vi "Autofocus-Broken.vi"(0 "controller in":refnum<k24>, 1 "AbortAutoFocus":bool, 5 "SafeMaxZ":dbl=86.0 format="%#_13g", 7 "InitialStepSize":dbl=0.1, 9 "Tolerance":dbl=0.005 format="%#_13g", 11 "error in (no error)":errorcluster) -> (4 "controller out":refnum<k24>, 6 "Image":T2(plugin-control), 8 "N_iterations":dbl, 10 "BestZvalue":dbl, 15 "error out":errorcluster)   [LabVIEW 2019]
uses:
  <vilib>/vision/NI_Vision_Development_Module.lvlib
  <vilib>/vision/driver/NI_Vision_Acquisition_Software.lvlib
  <vilib>/vision/driver/IMAQdx.llb/IMAQdx Buffer Number Mode.ctl
  <vilib>/Utility/error.llb/DialogType.ctl
  C:/Users/TTUHEP/Documents/LabVIEW/Other Models/2010/Bin/Aerotech.A3200.dll
  Other Models/2010/Bin/Aerotech.A3200.dll
  <vilib>/userDefined/High Color/IMAQdx.ctl
panel:
  out "ZvsSD":string
  in  "Camera":T1="cam1"
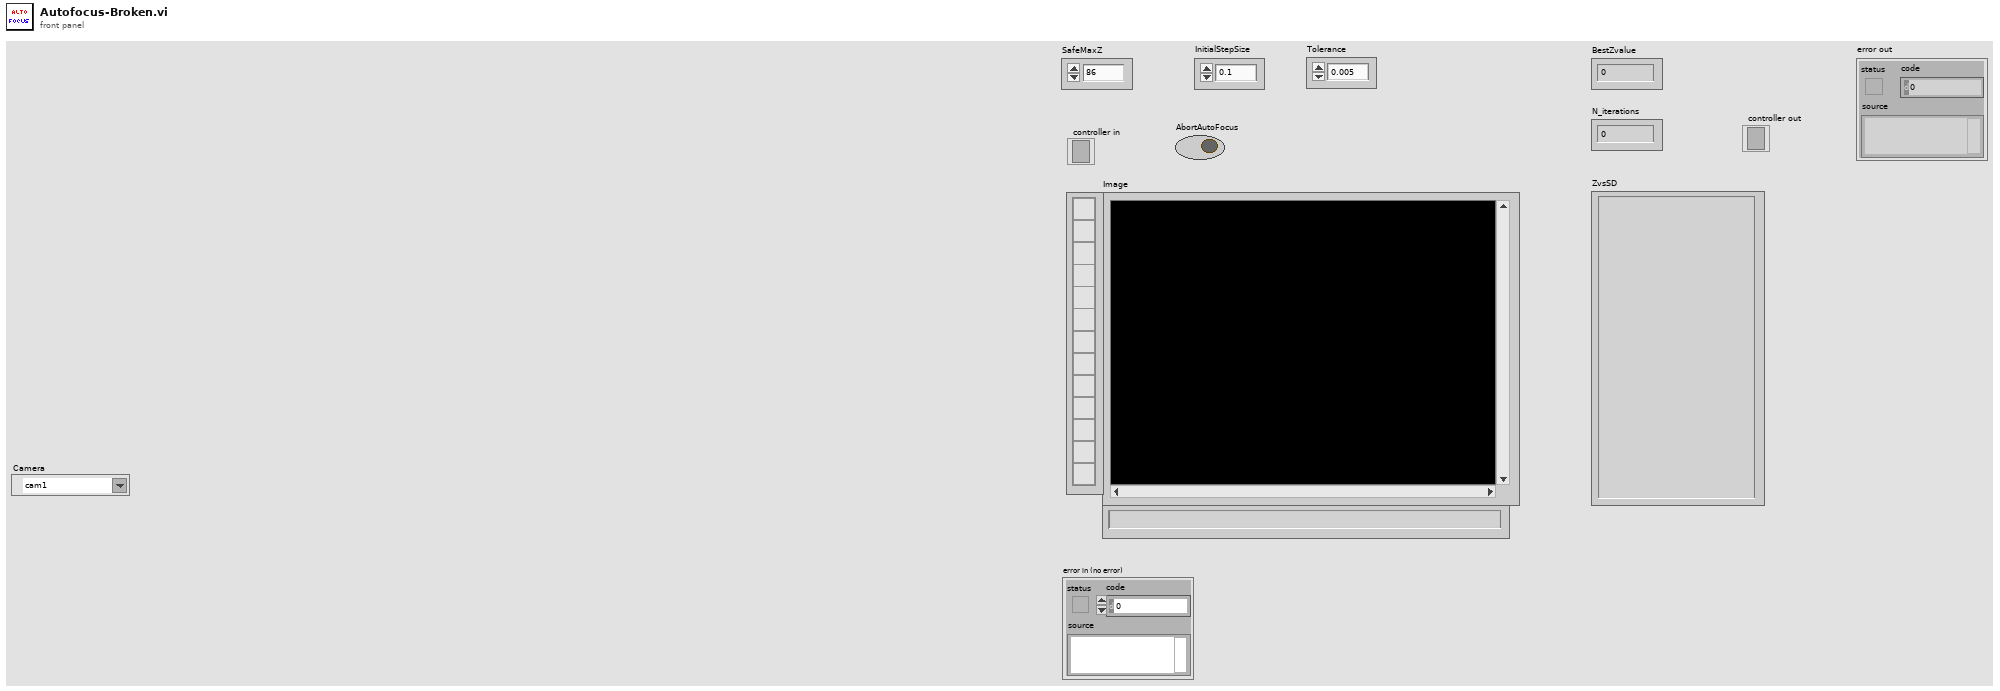
[diagram p1: front panel]
types:
  T1 = typedef "IMAQdx.ctl" = refnum<k21>
  T2 = typedef "IMAQ Image.ctl" = refnum<image>
  T3 = typedef "Image Type" = u32
  T4 = enum32{"Differentiation", "Gradient", "Prewitt", "Roberts", "Sigma", "Sobel"}
  T5 = typedef "NI_Vision_Acquisition_Software.lvlib/IMAQdx Buffer Number Mode.ctl" = enum32{"Next", "Last", "Buffer Number", "Every", "Last New"}
  T6 = typedef "DialogType.ctl" = u16
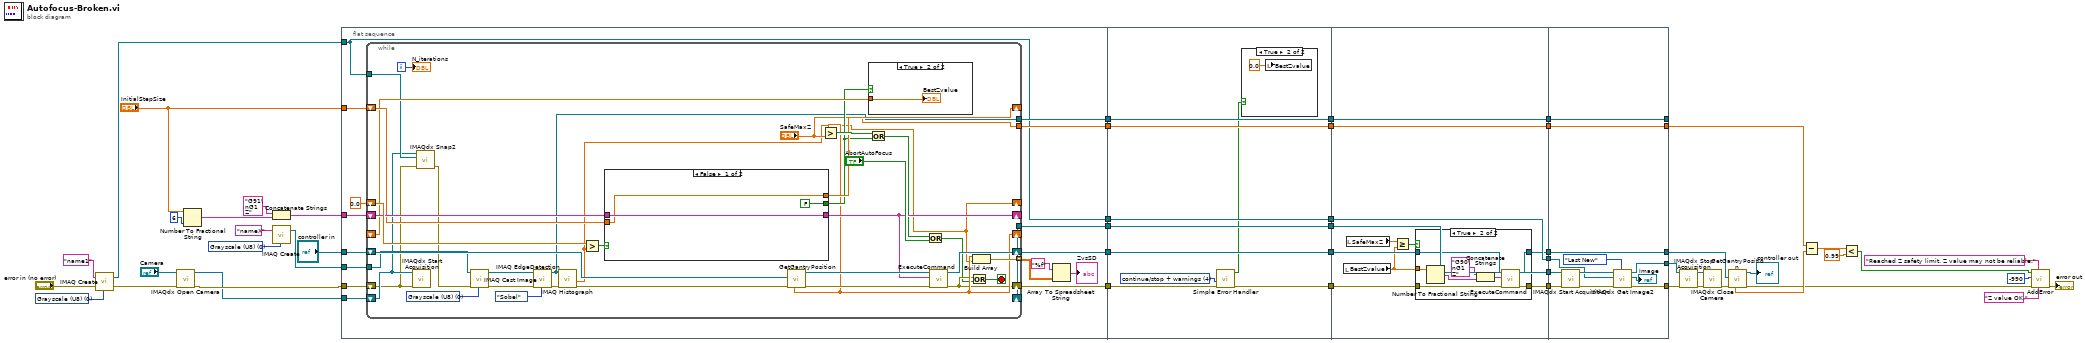
[diagram p0: block diagram]
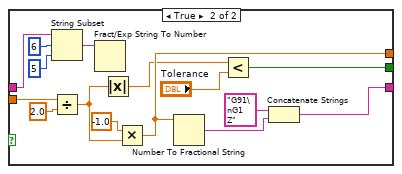
[diagram p3: hidden frame]
diagram:
  w26 = T3 0 items=["Grayscale (U8)", "Grayscale (I16)", "Grayscale (SGL)", "Complex (CSG)", "RGB (U32)", "HSL (U32)", "RGB (U64)", "Grayscale (U16)"] ("Image Type")
  w29 = T3 0 items=["Grayscale (U8)", "Grayscale (I16)", "Grayscale (SGL)", "Complex (CSG)", "RGB (U32)", "HSL (U32)", "RGB (U64)", "Grayscale (U16)"] ("Image Type")
  n1 = call "IMAQ Create"("Image Name"="name1" ("ImageName"), "Image Type"=w29, "error in (no error)"="error in (no error)") -> ("New Image"=w28:T2, "error out"=w31:errorcluster)  [unwired: 2 in]
  n2 = call <vilib>:"IMAQdx Open Camera.vi"("error in"=w31, "Session In"="Camera") -> ("error out"=w18:errorcluster, "Session Out"=w17:T1)  [unwired: 8 in]
  n3 = Number To Fractional String(number="InitialStepSize", precision (6)=i16 6) -> (F-format string=w47:string)  [unwired: 2 in]
  n4 = Concatenate Strings("G91\nG1 Z", w47) -> (w49:string)
  n5 = call "IMAQ Create"("Image Name"="nameX", "Image Type"=w26) -> ("New Image"=w13:T2)  [unwired: 3 in, 1 out]
  n6 = flat-sequence {
    tunnel: "controller in" -> [w68]
    tunnel: "InitialStepSize" -> [w66]
    tunnel: w49 -> [w65]
    tunnel: w18 -> [w64]
    tunnel: [w63] -> w12
    tunnel: [w62] -> w10
    tunnel: [w61] -> w8
    tunnel: [w60] -> w6
    tunnel: [w58] -> w4
    tunnel: w17 -> [w59]
    tunnel: w28 -> [w53]
    tunnel: [w53] -> w2
    tunnel: w13 -> [w54]
    tunnel: w12 -> [w132]
    tunnel: [w132] -> w11
    tunnel: w10 -> [w131]
    tunnel: [w131] -> w9
    tunnel: w8 -> [w127]
    tunnel: [w126] -> w7
    tunnel: w6 -> [w130]
    tunnel: [w130] -> w5
    tunnel: w4 -> [w129]
    tunnel: [w129] -> w3
    tunnel: w2 -> [w128]
    tunnel: [w128] -> w1
    tunnel: w11 -> [w140]
    tunnel: [w137] -> w24
    tunnel: w9 -> [w144]
    tunnel: [w144] -> w23
    tunnel: w7 -> [w139]
    tunnel: [w138] -> w22
    tunnel: w5 -> [w143]
    tunnel: [w143] -> w21
    tunnel: w3 -> [w142]
    tunnel: [w142] -> w20
    tunnel: w1 -> [w141]
    tunnel: [w141] -> w19
    tunnel: [w164] -> _
    tunnel: [w165] -> w35
    tunnel: [w166] -> w46
    tunnel: w24 -> [w166]
    tunnel: w23 -> [w165]
    tunnel: w22 -> [w156]
    tunnel: w21 -> [w164]
    tunnel: [w155] -> w34
    tunnel: [w158] -> w33
    tunnel: w20 -> [w160]
    tunnel: w19 -> [w159]
    frame #0 {
      n7 = while {
        shift-right: [w98] -> w63
        shift-left: w68 -> [w101]
        shift-right: [w75] -> w61
        shift-left: w64 -> [w70]
        shift-right: [w95] -> _
        shift-left: w65 -> [w94]
        shift-right: [w78] -> _
        shift-left: 0.0 -> [w97]
        shift-right: [w91] -> _
        shift-left: w66 -> [w90]
        shift-right: [w79] -> _
        shift-left: _ -> [w89]
        tunnel: ["SafeMaxZ"] -> w62
        tunnel: [w83] -> w60
        tunnel: w54 -> [w77]
        tunnel: [w76] -> w58
        tunnel: [w80] -> w55 mode=indexing
        shift-right: [w76] -> _
        shift-left: w59 -> [w71]
        tunnel: w53 -> [w72]
        i -> [w86]
        stop <- w73 stop-if-true
        w87 = T3 0 items=["Grayscale (U8)", "Grayscale (I16)", "Grayscale (SGL)", "Complex (CSG)", "RGB (U32)", "HSL (U32)", "RGB (U64)", "Grayscale (U16)"] ("Image Type")
        n8 = call <vilib>:"IMAQdx Start Acquisition.vi"("error in"=w70, "Session In"=w71) -> ()  [unwired: 8 in, 2 out]
        n9 = call <vilib>:"IMAQdx Snap2.vi"("error in"=w70, "Image In"=w72, "Session In"=w71) -> ("error out"=w69:errorcluster)  [unwired: 6 in, 2 out]
        n10 = call "IMAQ Cast Image"("Image Type"=w87, "error in (no error)"=w69, "Image Src"=w77) -> ("error out"=w81:errorcluster, "Image Dst Out"=w102:T2)  [unwired: 7 in]
        n11 = call "IMAQ EdgeDetection"("Method"=T4."Sobel", "error in (no error)"=w81, "Image Src"=w102) -> ("error out"=w104:errorcluster, "Image Dst Out"=w83:T2)  [unwired: 7 in]
        n12 = call "IMAQ Histograph"("error in (no error)"=w104, "Image"=w83) -> ("error out"=w84:errorcluster, "Standard  Deviation"=w78:sgl)  [unwired: 6 in, 2 out]
        n13 = Greater?(x=w97, y=w78) -> (0:w96:bool)
        n14 = case shown="False" w96 {
          tunnel: [w108 w122] -> w95
          tunnel: w94 -> [w108 w116]
          tunnel: [FALSE w117] -> w88
          tunnel: [w106 w112] -> w91
          tunnel: w90 -> [w106 w111]
          frame False {
          }
          frame True {
            n15 = String Subset(string=w116, offset (0)=6, length (rest)=5) -> (substring=w113:string)
            n16 = Divide(x=w111, y=2.0) -> (x/y=w110:dbl)
            n17 = Fract/Exp String To Number(string=w113) -> ()  [unwired: 3 in, 2 out]
            n18 = Absolute Value(x=w110) -> (abs(x)=w109:dbl)
            n19 = Multiply(x=-1.0, y=w110) -> (x*y=w112:dbl)
            n20 = Number To Fractional String(number=w112) -> (F-format string=w121:string)  [unwired: 3 in]
            n21 = Less?(x=w109, y="Tolerance") -> (x < y?=w117:bool)
            n22 = Concatenate Strings("G91\nG1 Z", w121) -> (w122:string)
          }
        }
        n23 = call "GetGantryPosition.vi"("error in (no error)"=w84, "Controller In"=w101) -> ("error out"=w100:errorcluster, "controller out"=w99:refnum<k24>, "Position Z"=w79:dbl)  [unwired: 3 in, 4 out]
        n24 = Greater?(x=w79, y="SafeMaxZ") -> (0:w93:bool)
        n25 = case shown="True" w88 {
          tunnel: w89 -> [_ w105]
          frame False {
          }
          frame True {
            "BestZvalue" <- w105
          }
        }
        n26 = Or(x=w93, y=w88) -> (x .or. y?=w92:bool)
        n27 = Or(x=w92, y="AbortAutoFocus") -> (x .or. y?=w74:bool)
        n28 = call "ExecuteCommand.vi"("error in (no error)"=w100, "Command Code"=w95, "controller in"=w99) -> ("error out"=w75:errorcluster, "controller out"=w98:refnum<k24>)  [unwired: 6 in, 1 out]
        n29 = Or(x=w75, y=w74) -> (x .or. y?=w73:bool)
        n30 = Build Array(w79, w78) -> (w80:dbl[])
        "N_iterations" <- w86
      }
      n31 = Array To Spreadsheet String(array=w55, 3:"%f" ("format string")) -> (spreadsheet string=→"ZvsSD":string)  [unwired: 1 in]
    }
    frame #1 {
      w124 = T6 4 items=["no dialog", "OK message", "continue or stop message", "OK message + warnings", "continue/stop + warnings"] ("type of dialog (OK msg:1)")
      n32 = call <vilib>:"Simple Error Handler.vi"("type of dialog (OK msg:1)"=w124, "error in (no error)"=w127) -> ("error?"=w125:bool, "error out"=w126:errorcluster)  [unwired: 3 in, 3 out]
      n33 = case shown="True" w125 {
        frame False {
        }
        frame True {
          n34 = local write "BestZvalue"(0.0 ("BestZvalue")) -> ()
        }
      }
    }
    frame #2 {
      n35 = local read "BestZvalue"() -> (w135:dbl)
      n36 = local read "SafeMaxZ"() -> (w136:dbl)
      n37 = Greater Or Equal?(x=w136, y=w135) -> (x >= y?=w134:bool)
      n38 = case shown="True" w134 {
        tunnel: w140 -> [w146 w154]
        tunnel: w139 -> [w145 w153]
        tunnel: [w145 w149] -> w138
        tunnel: [w146 w148] -> w137
        tunnel: w135 -> [_ w147]
        frame False {
        }
        frame True {
          n39 = Number To Fractional String(number=w147) -> (F-format string=w152:string)  [unwired: 3 in]
          n40 = Concatenate Strings("G90\nG1 Z", w152) -> (w150:string)
          n41 = call "ExecuteCommand.vi"("error in (no error)"=w153, "Command Code"=w150, "controller in"=w154) -> ("error out"=w149:errorcluster, "controller out"=w148:refnum<k24>)  [unwired: 6 in, 1 out]
        }
      }
    }
    frame #3 {
      n42 = call <vilib>:"IMAQdx Start Acquisition.vi"("error in"=w156, "Session In"=w160) -> ("error out"=w162:errorcluster, "Session Out"=w163:T1)  [unwired: 8 in]
      n43 = call <vilib>:"IMAQdx Get Image2.vi"("Buffer Number Mode (Next)"=IMAQdx_Buffer_Number_Mode."Last New", "error in"=w162, "Image In"=w159, "Session In"=w163) -> ("error out"=w155:errorcluster, "Image Out"=→"Image":T2, "Session Out"=w158:T1)  [unwired: 4 in, 1 out]
    }
  }
  n44 = call <vilib>:"IMAQdx Stop Acquisition.vi"("error in"=w34, "Session In"=w33) -> ("error out"=w15:errorcluster, "Session Out"=w16:T1)  [unwired: 8 in]
  n45 = call <vilib>:"IMAQdx Close Camera.vi"("error in"=w15, "Session In"=w16) -> ("error out"=w14:errorcluster)  [unwired: 9 in]
  n46 = call "GetGantryPosition.vi"("error in (no error)"=w14, "Controller In"=w46) -> ("error out"=w39:errorcluster, "controller out"=→"controller out":refnum<k24>, "Position Z"=w44:dbl)  [unwired: 3 in, 4 out]
  n47 = Subtract(x=w35, y=w44) -> (x-y=w43:dbl)
  n48 = Less?(x=w43, y=0.99) -> (x < y?=w41:bool)
  n49 = call "AddError.vi"("NoErrorMessage"="Z value OK.", "ErrorMessage"="Reached Z safety limit. Z value may not be reliable.", "error in"=w39, "code"=-990, "Error?"=w41) -> ("Error out"=→"error out":errorcluster)  [unwired: 6 in]
